vi "Close.vi"(8 "error in (no error)":errorcluster, 11 "Server Port in":u16) -> (0 "error out":errorcluster, 1 "ms Elapsed":u32)   [LabVIEW 2021, in "HttpServer.lvlib"]
uses:
  HttpServer.lvlib
  TypeDefs/Action.ctl
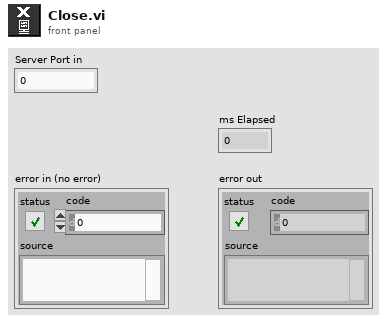
[diagram p1: front panel]
types:
  T1 = typedef "HttpServer.lvlib/Action.ctl" = enum8{"noop", "add", "get", "set", "remove"}
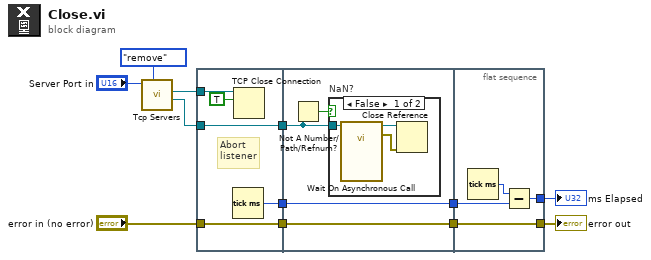
[diagram p0: block diagram]
diagram:
  n1 = call "Tcp Servers.vi"("Action"=Action."remove", "Server Port in"="Server Port in") -> ("VI out"=w1:refnum<vi>, "Connection out"=w10:refnum<k5>)  [unwired: 6 in, 2 out]
  n2 = flat-sequence {
    tunnel: [w16] -> w7
    tunnel: [w15] -> w6
    tunnel: [w14] -> w3
    tunnel: w10 -> [w17]
    tunnel: "error in (no error)" -> [w16]
    tunnel: w1 -> [w15]
    tunnel: w7 -> [w21]
    tunnel: w6 -> [w20]
    tunnel: [w21] -> w5
    tunnel: [w18] -> w4
    tunnel: w3 -> [w18]
    tunnel: [w28] -> w9
    tunnel: w5 -> [w28]
    tunnel: w4 -> [w26]
    tunnel: [w25] -> w2
    frame #0 {
      # "Abort\nlistener"
      n3 = Tick Count (ms)() -> (millisecond timer value=w14:u32)
      n4 = TCP Close Connection(connection ID=w17, abort (F)=TRUE) -> ()  [unwired: 1 in, 2 out]
    }
    frame #1 {
      n5 = Not A Number/Path/Refnum?(number/path/refnum=w20) -> (NaN/Path/Refnum?=w19:bool)
      n6 = case "NaN?" shown="False" w19 {
        tunnel: w20 -> [w24 _]
        frame False {
          n7 = call-by-ref "Wait On Asynchronous Call"(reference=w24) -> (reference out=w23:refnum<vi>, error out=w22:errorcluster)  [unwired: 13 in]
          n8 = Close Reference(reference=w23, error in (no error)=w22) -> ()  [unwired: 1 out]
        }
        frame True {
        }
      }
    }
    frame #2 {
      n9 = Tick Count (ms)() -> (millisecond timer value=w27:u32)
      n10 = Subtract(x=w27, y=w26) -> (x-y=w25:u32)
    }
  }
  "error out" <- w9
  "ms Elapsed" <- w2
